vi "Request Data (Synchronous).vi"(4 "Ignore Past Updates? (F)":bool, 8 "error in (no error)":errorcluster, 9 "Topic Name (Use Control Text)":string, 10 "Type":variant, 11 "IObserver in":refnum<class "IObserver.lvclass">) -> (0 "error out":errorcluster, 3 "IObserver out":refnum<class "IObserver.lvclass">)   [LabVIEW 2015, in "IObserver.lvlib" / "IObserver.lvclass"]
doc: "<License>\nCopyright © 2017 Composed Systems, LLC | All rights reserved\nwww.composed.io\n\nAuthor: Ethan Stern <ethan.stern@composed.io>\n\nThis software is provided \"AS IS\" WITHOUT WARRANTIES, either express or implied, AND IS FOR EDUCATIONAL PURPOSES ONLY.\n</License>"
uses:
  IObserver.lvclass
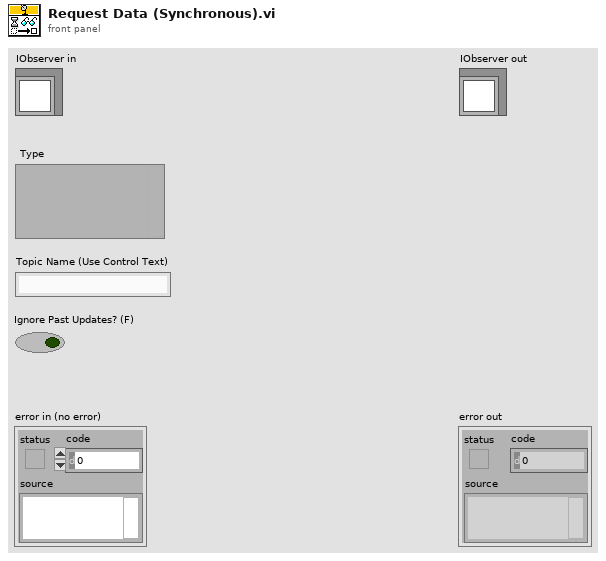
[diagram p1: front panel]
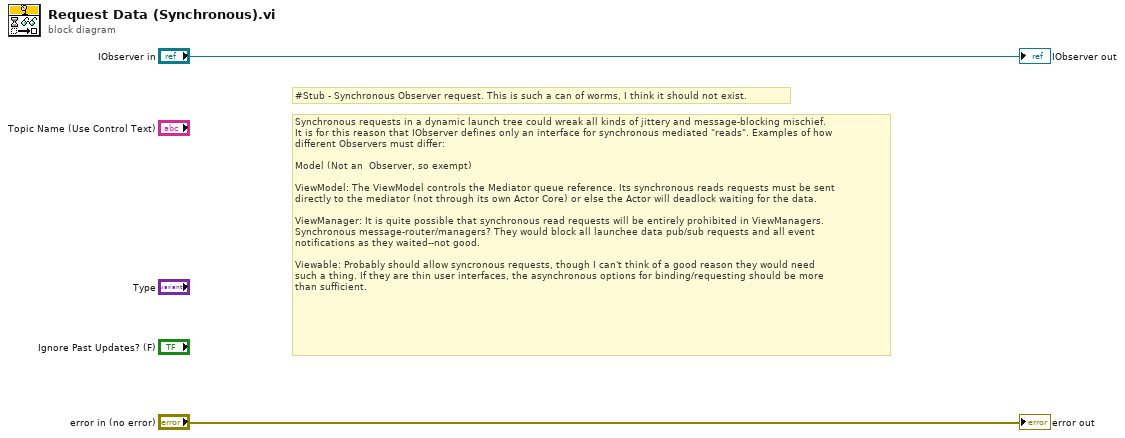
[diagram p0: block diagram]
diagram:
  # "#Stub - Synchronous Observer request. This is such a can of worms, I think it should not exist."
  # "Synchronous requests in a dynamic launch tree could wreak all kinds of jittery and message-blocking mischief.\nIt is for this reason that IObserver defines only an interface for synchronous mediated \"reads\". Examples of how\ndifferent Observers must differ:\n\nModel (Not an  Observer, so exempt)\n\nViewModel: The ViewModel controls the Mediator queue reference. Its synchronous reads requests must be sent\ndirectly to the mediator (not through its own Actor Core) or else the Actor will deadlock waiting for the data.\n\nViewManager: It is quite possible that synchronous read requests will be entirely prohibited in ViewManagers.\nSynchronous message-router/managers? They would block all launchee data pub/sub requests and all event\nnotifications as they waited--not good.\n\nViewable: Probably should allow syncronous requests, though I can't think of a good reason they would need\nsuch a thing. If they are thin user interfaces, the asynchronous options for binding/requesting should be more\nthan sufficient."
  "error out" <- "error in (no error)"
  "IObserver out" <- "IObserver in"
